vi "InvSymmetricalComponents_src.vi"(0 "zero":T1, 5 "positive":T1, 7 "negative":T1) -> (4 "a":T1, 6 "b":T1, 8 "c":T1)   [LabVIEW 2017]
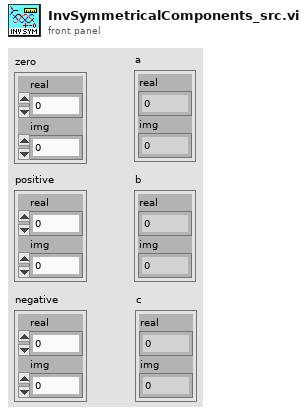
[diagram p1: front panel]
types:
  T1 = typedef "ComplexSGL" = cluster{"real":sgl, "img":sgl}
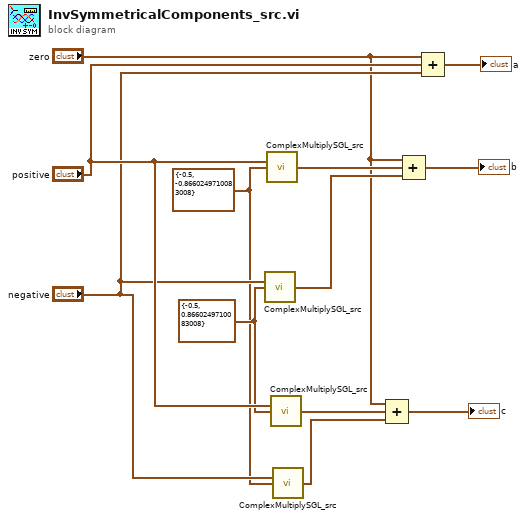
[diagram p0: block diagram]
diagram:
  w8 = T1 {"real"=-0.5, "img"=0.866025} ("Y")
  w6 = T1 {"real"=-0.5, "img"=-0.866025} ("Y")
  n1 = call "ComplexMultiplySGL_src.vi"("X"="negative", "Y"=w8) -> ("Z"=w10:T1)  [unwired: 13 in]
  n2 = call "ComplexMultiplySGL_src.vi"("X"="positive", "Y"=w6) -> ("Z"=w11:T1)  [unwired: 13 in]
  n3 = call "ComplexMultiplySGL_src.vi"("X"="positive", "Y"=w8) -> ("Z"=w4:T1)  [unwired: 13 in]
  n4 = call "ComplexMultiplySGL_src.vi"("X"="negative", "Y"=w6) -> ("Z"=w3:T1)  [unwired: 13 in]
  n5 = Compound Arithmetic op=ADD("zero", w4, w3) -> (→"c":T1)
  n6 = Compound Arithmetic op=ADD("zero", w11, w10) -> (→"b":T1)
  n7 = Compound Arithmetic op=ADD("zero", "positive", "negative") -> (→"a":T1)
